vi "Preprocess Variant.vi"(11 "Variant":variant) -> (2 "Array":bool[](array[boolean]), 3 "Array 2":string[](array[string]))   [LabVIEW 2019, in "JSON-Schema.lvlib"]
uses:
  JSON-Schema.lvlib
  <vilib>/Utility/Data Type/NI_Data Type.lvlib
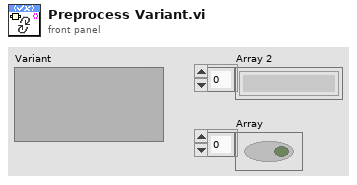
[diagram p1: front panel]
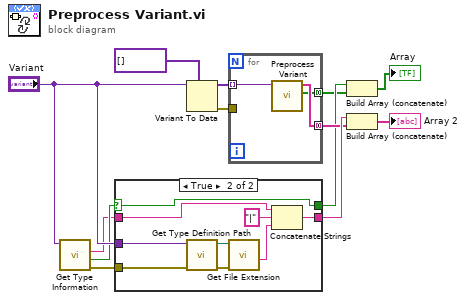
[diagram p0: block diagram]
diagram:
  n1 = call <vilib>:"Get Type Information.vi"("variant"="Variant") -> ("error out"=w8:errorcluster, "type definition"=w9:bool, "name"=w1:string)  [unwired: 6 in, 2 out]
  n2 = case shown="True" w9 {
    selector: w9 -> [w15 w20]
    tunnel: w8 -> [_ w22]
    tunnel: "Variant" -> [_ w21]
    tunnel: [w14 w19] -> w7
    tunnel: [w15 w20] -> w5
    tunnel: w1 -> [w14 w18]
    frame False {
    }
    frame True {
      n3 = call <vilib>:"Get Type Definition Path.vi"("error in (no error)"=w22, "variant"=w21) -> ("error out"=w23:errorcluster, "type definition path"=w24:path)  [unwired: 8 in]
      n4 = call <vilib>:"Get File Extension.vi"("error in (no error)"=w23, "file"=w24) -> ("filename without extension"=w16:string)  [unwired: 5 in, 4 out]
      n5 = Concatenate Strings(w18, "|" ("string"), w16) -> (w19:string)
    }
  }
  n6 = Variant To Data(type=variant[] [], Variant="Variant") -> (data=w12:variant[], error out=w13:errorcluster)  [unwired: 1 in]
  n7 = for {
    tunnel: w12 -> [w27] mode=indexing
    tunnel: w13 -> [_]
    tunnel: [w26] -> w6 mode=concatenating
    tunnel: [w25] -> w4 mode=concatenating
    n8 = call "Preprocess Variant.vi"("Variant"=w27) -> ("Array"=w25:bool[], "Array 2"=w26:string[])  [unwired: 9 in]
  }
  n9 = Build Array (concatenate)(w5, w4) -> (→"Array":bool[])
  n10 = Build Array (concatenate)(w7, w6) -> (→"Array 2":string[])
